vi "writeread.vi"(0 "VISA resource input":refnum<visa-resource-name>, 1 "Read Delay":dbl, 2 "write buffer":string, 3 "error in (no error)":errorcluster, 4 "Max Read Buffer":i32=100) -> (6 "VISA resource out":refnum<visa-resource-name>, 7 "Response 2":string, 9 "error out":errorcluster)   [LabVIEW 2018]
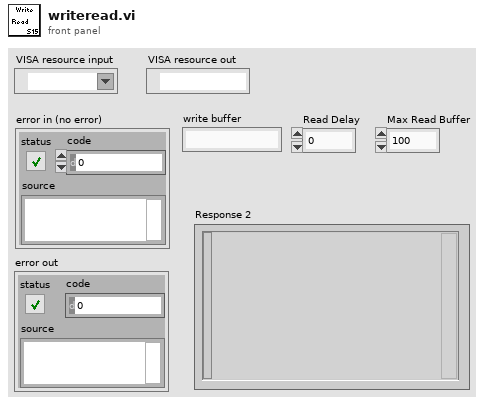
[diagram p1: front panel]
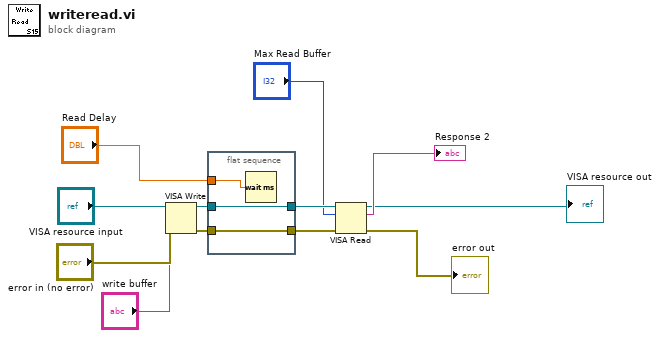
[diagram p0: block diagram]
diagram:
  n1 = VISA Write(VISA resource name="VISA resource input", write buffer="write buffer", error in (no error)="error in (no error)") -> (VISA resource name out=w11:refnum<visa-resource-name>, error out=w12:errorcluster)  [unwired: 1 out]
  n2 = flat-sequence {
    tunnel: w12 -> [w14]
    tunnel: [w14] -> w10
    tunnel: w11 -> [w13]
    tunnel: [w13] -> w9
    tunnel: "Read Delay" -> [w15]
    frame #0 {
      n3 = Wait (ms)(milliseconds to wait=w15) -> ()  [unwired: 1 out]
    }
  }
  n4 = VISA Read(VISA resource name=w9, byte count="Max Read Buffer", error in (no error)=w10) -> (VISA resource name out=→"VISA resource out":refnum<visa-resource-name>, read buffer=→"Response 2":string, error out=→"error out":errorcluster)  [unwired: 1 out]
